vi "Router - Data Integrity -  Ch Mapping.vi"() -> ()   [LabVIEW 2016]
uses:
  XML Cluster.ctl
  Node Properties.ctl
  <vilib>/Utility/error.llb/DialogType.ctl
  <vilib>/pximc/Initialize Writer Session (DBL).vi
  <vilib>/pximc/Connect (DBL).vi
  <vilib>/pximc/Initialize Reader Session (DBL).vi
  <vilib>/pximc/Acquire Read Region (DBL).vi
  <vilib>/pximc/Acquire Write Region (DBL).vi
  <vilib>/pximc/nipximc.lvlib
  <resource>/objmgr/pximc.rc
panel:
  out "Waveform Chart":T1(graph)
  out "Stopped":bool
  in  "Configuration Properties":T2={"Node Properties"=[{"Resource Name"="PXI1Slot2", "Slave IP Address"="", "Node ID"=1, "Node # Channels"=2, "Data Importing Nodes"=[]}, {"Resource Name"="PXI1Slot2", "Slave IP Address"="", "Node ID"=2, "Node # Channels"=2, "Data Importing Nodes"=[]}], "Connection Timeout (s)"=60.0, "Readers Buffer Size"=250000}
  in  "Stop Button":bool
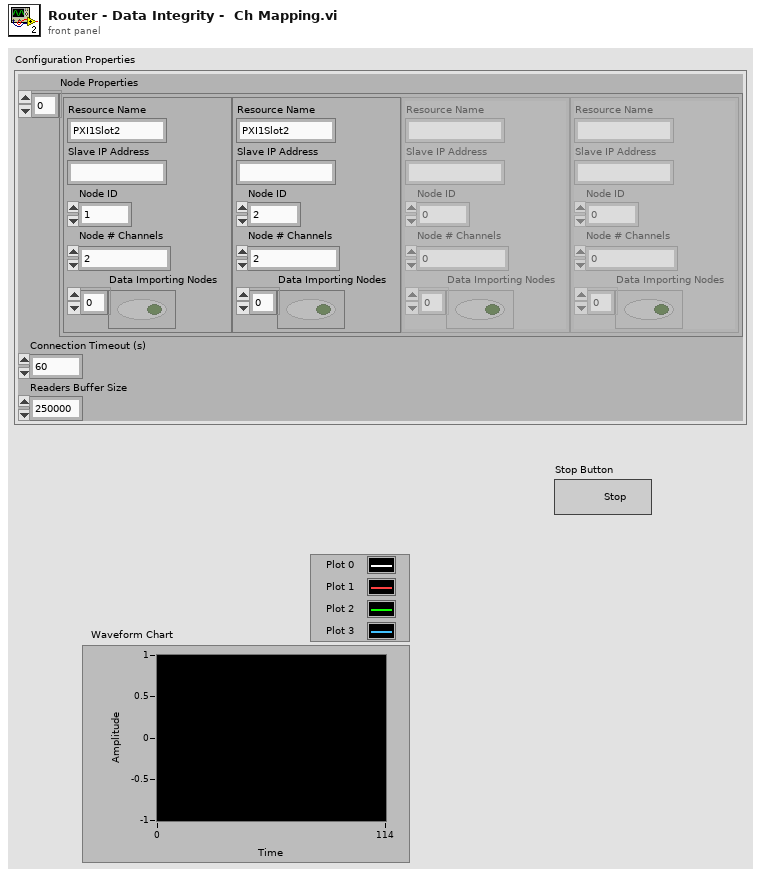
[diagram p1: front panel]
types:
  T1 = cluster{"[0]":dbl, "[1]":dbl, "[2]":dbl, "[3]":dbl, "[4]":dbl, "[5]":dbl, "[6]":dbl, "[7]":dbl, "[8]":dbl}
  T2 = typedef "XML Cluster.ctl" = cluster{"Node Properties":T3[], "Connection Timeout (s)":dbl, "Readers Buffer Size":u32}
  T3 = typedef "Node Properties.ctl" = cluster{"Resource Name":string, "Slave IP Address":string, "Node ID":u16, "Node # Channels":u32, "Data Importing Nodes":bool[]}
  T4 = typedef "DialogType.ctl" = u16
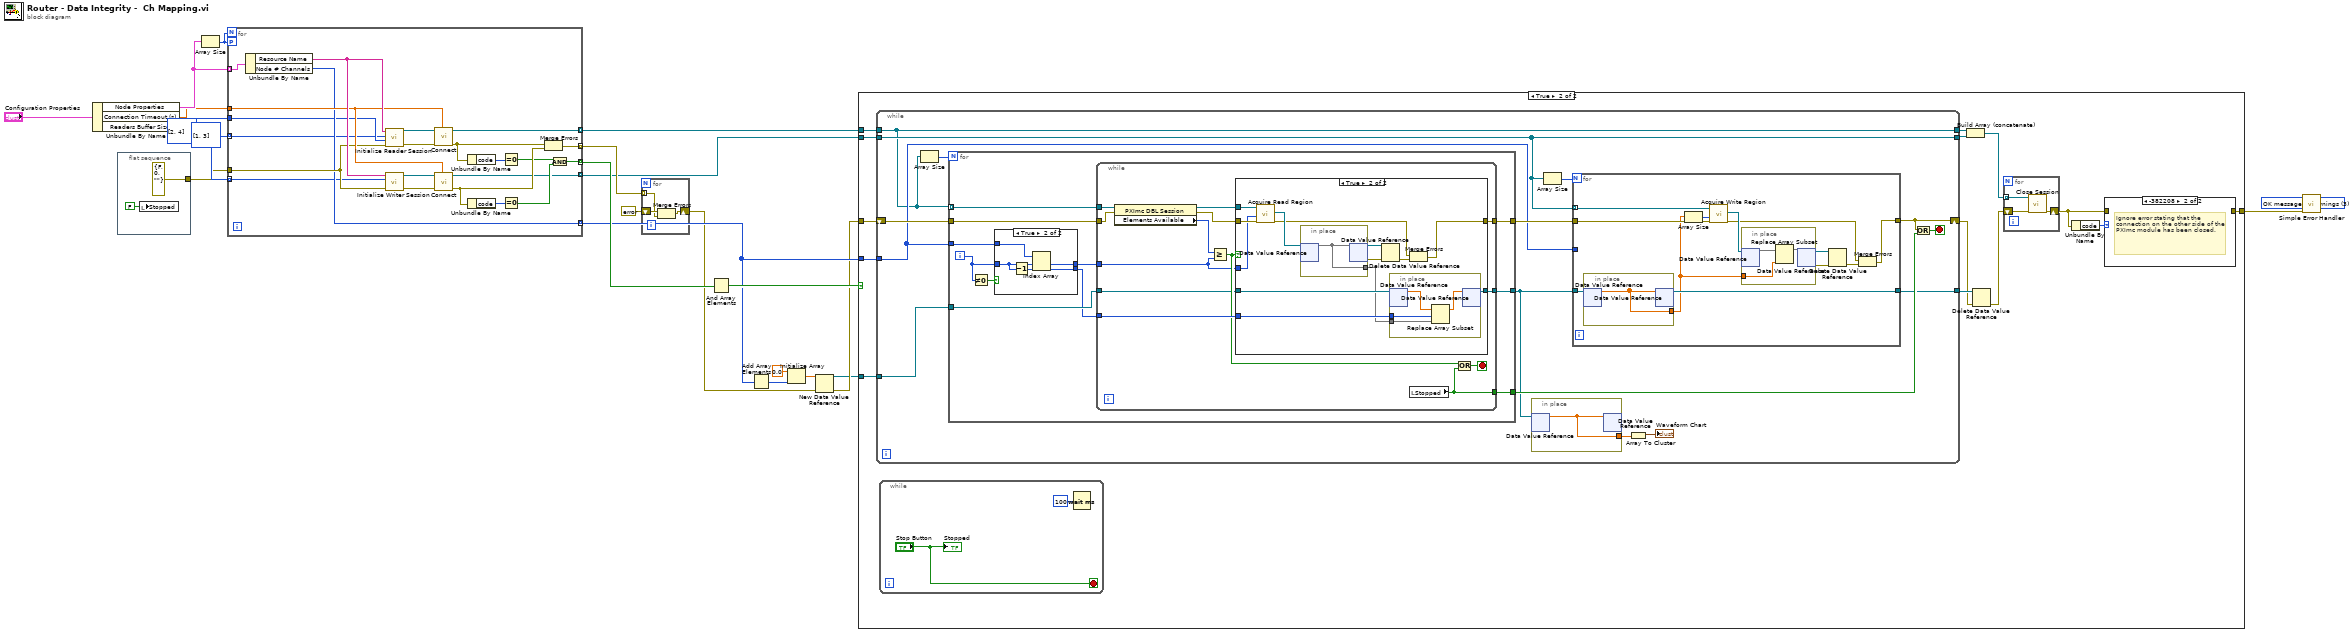
[diagram p0: block diagram]
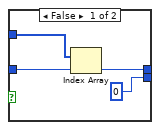
[diagram p4: hidden frame]
diagram:
  w11 = T4 3 items=["no dialog", "OK message", "continue or stop message", "OK message + warnings", "continue/stop + warnings"] ("type of dialog (OK msg:1)")
  n1 = Unbundle By Name("Configuration Properties") -> ("Node Properties"=w22:T3[], "Connection Timeout (s)"=w20:dbl, "Readers Buffer Size"=w10:u32)
  n2 = flat-sequence {
    tunnel: [errorcluster {"status"=FALSE, "code"=0, "source"=""} ("error constant")] -> w1
    frame #0 {
      n3 = local write "Stopped"(FALSE ("Stopped")) -> ()
    }
  }
  n4 = Array Size(array=w22) -> (size(s)=w21:i32)
  n5 = for {
    N: w21 -> [_]
    tunnel: w22 -> [w47] mode=indexing
    workers-P: w21 -> [_]
    tunnel: w20 -> [w43]
    tunnel: w1 -> [w41]
    tunnel: [w33] -> w19 mode=indexing
    tunnel: [w32] -> w14 mode=indexing
    tunnel: [w31] -> w15 mode=indexing
    tunnel: [w30] -> w13 mode=indexing
    tunnel: [w29] -> w17 mode=indexing
    tunnel: w10 -> [w28]
    tunnel: i32[] [2, 4] -> [w27] mode=indexing
    tunnel: i32[] [1, 3] -> [w26] mode=indexing
    n6 = Unbundle By Name(w47) -> ("Resource Name"=w46:string, "Node # Channels"=w30:u32)
    n7 = call-poly <vilib>:"Initialize Reader Session.vi"("error in (no error)"=w41, "buffer size"=w28, "writer's connection id (1)"=w26, "interface"=w46) -> ("error out"=w44:errorcluster, "session out"=w45:refnum<k21>)  [unwired: 6 in]
    n8 = call-poly <vilib>:"Initialize Writer Session.vi"("error in (no error)"=w41, "connection id (1)"=w27, "interface"=w46) -> ("error out"=w42:errorcluster, "session out"=w38:refnum<k21>)  [unwired: 7 in]
    n9 = call-poly <vilib>:"Connect.vi"("timeout in seconds (-1)"=w43, "error in (no error)"=w44, "session in"=w45) -> ("error out"=w39:errorcluster, "session out"=w31:refnum<k21>)  [unwired: 7 in]
    n10 = call-poly <vilib>:"Connect.vi"("timeout in seconds (-1)"=w43, "error in (no error)"=w42, "session in"=w38) -> ("error out"=w36:errorcluster, "session out"=w32:refnum<k21>)  [unwired: 7 in]
    n11 = Unbundle By Name(w39) -> ("code"=w40:i32)
    n12 = Unbundle By Name(w36) -> ("code"=w37:i32)
    n13 = Equal To 0?(x=w40) -> (x = 0?=w35:bool)
    n14 = Equal To 0?(x=w37) -> (x = 0?=w34:bool)
    n15 = Merge Errors(w39, w36) -> (w29:errorcluster)
    n16 = And(x=w35, y=w34) -> (x .and. y?=w33:bool)
  }
  n17 = for {
    tunnel: w17 -> [w49] mode=indexing
    shift-right: [w48] -> w4
    shift-left: errorcluster {"status"=FALSE, "code"=0, "source"=""} ("error constant") -> [w50]
    n18 = Merge Errors(w50, w49) -> (w48:errorcluster)
  }
  n19 = And Array Elements(Boolean array=w19) -> (logical AND=w18:bool)
  n20 = Add Array Elements(numeric array=w13) -> (sum=w5:u32)
  n21 = Initialize Array(0.0 ("element"), w5) -> (w7:dbl[])
  n22 = New Data Value Reference(data value=w7, error in=w4) -> (data value reference=w2:refnum<data-value>, error out=w3:errorcluster)
  n23 = case shown="True" w18 {
    tunnel: w15 -> [_ w65]
    tunnel: w14 -> [_ w64]
    tunnel: [w51 w58] -> w12
    tunnel: w3 -> [w51 w57]
    tunnel: w13 -> [_ w56]
    tunnel: w2 -> [_ w55]
    frame False {
    }
    frame True {
      n24 = while {
        tunnel: w65 -> [w68]
        tunnel: w64 -> [w74]
        shift-right: [w73] -> w53
        shift-left: w57 -> [w76]
        tunnel: [w68] -> w62
        tunnel: [w74] -> w61
        tunnel: w56 -> [w69]
        tunnel: w55 -> [w77]
        tunnel: [w75] -> w54
        stop <- w78 stop-if-true
        n25 = Array Size(array=w68) -> (size(s)=w67:i32)
        n26 = for {
          N: w67 -> [_]
          tunnel: w68 -> [w91] mode=indexing
          tunnel: [w90] -> w79
          tunnel: w77 -> [w89]
          tunnel: w69 -> [w83]
          tunnel: [w88] -> w72
          tunnel: w76 -> [w87]
          tunnel: [w86] -> w80
          i -> [w84]
          n27 = Not Equal To 0?(x=w84) -> (x != 0?=w85:bool)
          n28 = case shown="True" w85 {
            tunnel: w84 -> [w126 w132]
            tunnel: [w127 w130] -> w82
            tunnel: [0 w131] -> w81
            tunnel: w83 -> [w125 w129]
            frame False {
              n29 = Index Array(array=w125, index=w126) -> (element=w127:u32)
            }
            frame True {
              n30 = Decrement(x=w132) -> (x-1=w133:i32)
              n31 = Index Array(array=w129, index #1=w132, index #2=w133) -> (element #1=w130:u32, element #2=w131:u32)
            }
          }
          n32 = while {
            tunnel: w91 -> [w103]
            tunnel: w87 -> [w100]
            tunnel: [w104] -> w86
            tunnel: [w98] -> w88
            tunnel: w81 -> [w97]
            tunnel: [w92] -> w90
            tunnel: w89 -> [w94]
            tunnel: w82 -> [w93]
            stop <- w95 stop-if-true
            n33 = property class="PXImc DBL Session"(reference=w103, error in=w100) -> (reference out=w101:refnum<k21>, error out=w99:errorcluster, "Elements Available"=w102:u64)
            n34 = Greater Or Equal?(x=w102, y=w93) -> (x >= y?=w96:bool)
            n35 = case shown="True" w96 {
              tunnel: w99 -> [w106 w118]
              tunnel: [w106 w112] -> w104
              tunnel: w101 -> [_ w117]
              tunnel: w97 -> [_ w111]
              tunnel: [w105 w108] -> w98
              tunnel: w93 -> [_ w110]
              tunnel: w94 -> [w105 w109]
              frame False {
              }
              frame True {
                n36 = call-poly <vilib>:"Acquire Read Region.vi"("error in (no error)"=w118, "number of elements"=w110, "session in"=w117) -> ("error out"=w113:errorcluster, "read region reference"=w119:refnum<data-value>)  [unwired: 5 in, 2 out]
                n37 = in-place {
                  in-place-border: [w124] -> w107
                  n38 = in-place-dvr #1(w119) -> (w124:dbl[])  [unwired: 1 out]
                  n39 = in-place-dvr #1(w124) -> (w116:refnum<data-value>, w115:errorcluster)
                }
                n40 = Delete Data Value Reference(data value reference=w116, error in=w115) -> (error out=w114:errorcluster)  [unwired: 1 out]
                n41 = in-place {
                  in-place-border: w111 -> [w123]
                  in-place-border: w107 -> [w120]
                  n42 = in-place-dvr #2(w109) -> (w122:dbl[])  [unwired: 1 out]
                  n43 = Replace Array Subset(array=w122, new element=w120, index=w123) -> (w121:dbl[])
                  n44 = in-place-dvr #2(w121) -> (w108:refnum<data-value>)  [unwired: 1 out]
                }
                n45 = Merge Errors(w113, w114) -> (w112:errorcluster)
              }
            }
            n46 = local read "Stopped"() -> (w92:bool)
            n47 = Or(x=w96, y=w92) -> (x .or. y?=w95:bool)
          }
        }
        n48 = in-place {
          in-place-border: [w134] -> w70
          n49 = in-place-dvr #3(w72) -> (w134:dbl[])  [unwired: 1 out]
          n50 = in-place-dvr #3(w134) -> ()  [unwired: 2 out]
        }
        n51 = Array Size(array=w74) -> (size(s)=w66:i32)
        n52 = for {
          N: w66 -> [_]
          tunnel: w74 -> [w141] mode=indexing
          tunnel: w69 -> [_]
          tunnel: w72 -> [w146]
          tunnel: [w145] -> w75
          tunnel: w80 -> [w140]
          tunnel: [w137] -> w73
          n53 = in-place {
            in-place-border: [w147] -> w136
            n54 = in-place-dvr #4(w146) -> (w147:dbl[])  [unwired: 1 out]
            n55 = in-place-dvr #4(w147) -> (w145:refnum<data-value>)  [unwired: 1 out]
          }
          n56 = Array Size(array=w136) -> (size(s)=w135:i32)
          n57 = call-poly <vilib>:"Acquire Write Region.vi"("error in (no error)"=w140, "number of elements"=w135, "session in"=w141) -> ("error out"=w138:errorcluster, "write region reference"=w139:refnum<data-value>)  [unwired: 5 in, 2 out]
          n58 = in-place {
            in-place-border: w136 -> [w148]
            n59 = in-place-dvr #5(w139) -> (w150:dbl[])  [unwired: 1 out]
            n60 = Replace Array Subset(array=w150, new element=w148) -> (w149:dbl[])  [unwired: 1 in]
            n61 = in-place-dvr #5(w149) -> (w142:refnum<data-value>, w144:errorcluster)
          }
          n62 = Delete Data Value Reference(data value reference=w142, error in=w144) -> (error out=w143:errorcluster)  [unwired: 1 out]
          n63 = Merge Errors(w138, w143) -> (w137:errorcluster)
        }
        n64 = Array To Cluster(array=w70) -> (cluster=→"Waveform Chart":T1)
        n65 = Or(x=w73, y=w79) -> (x .or. y?=w78:bool)
      }
      n66 = while {
        stop <- "Stop Button" stop-if-true
        n67 = Wait (ms)(milliseconds to wait=u32 100) -> ()  [unwired: 1 out]
        "Stopped" <- "Stop Button"
      }
      n68 = Build Array (concatenate)(w62, w61) -> (w60:refnum<k21>[])
      n69 = Delete Data Value Reference(data value reference=w54, error in=w53) -> (error out=w52:errorcluster)  [unwired: 1 out]
      n70 = for {
        tunnel: w60 -> [w153] mode=indexing
        shift-right: [w151] -> w59
        shift-left: w52 -> [w152]
        n71 = call <vilib>:"Close Session.vi"("error in (no error)"=w152, "session in"=w153) -> ("error out"=w151:errorcluster)  [unwired: 9 in]
      }
      n72 = Unbundle By Name(w59) -> ("code"=w63:i32)
      n73 = case shown="-382208" w63 {
        tunnel: w59 -> [w154 _]
        tunnel: [w154 _] -> w58
        frame 0, Default {
        }
        frame -382208 {
          # "Ignore error stating that the connection on the other side of the PXImc module has been closed."
        }
      }
    }
  }
  n74 = call <vilib>:"Simple Error Handler.vi"("type of dialog (OK msg:1)"=w11, "error in (no error)"=w12) -> ()  [unwired: 3 in, 5 out]
